vi "Dictionary Get Values.vi"(7 "lock dictionary? (FALSE)":bool, 8 "error in":errorcluster, 11 "dictionary":T1) -> (0 "error out":errorcluster, 2 "values":variant[](array[variant]), 3 "dictionary out":T1)   [LabVIEW 2009]
doc: "Returns all of the values within the dictionary. \n\n<B>lock dictionary</B> will lock the dictionary, preventing dictionary modifications until it is unlocked. Locking a dictionary is useful when the values of keys store compound data, which might be modified in multiple locations. The dictionary may be unlocked using the <B>unlock dictionary</B> input of the <B>Update Dictionary</B> function."
uses:
  Dictionary Object RefNum.ctl
  Dictionary Object RefNum - Enum.ctl
panel:
  # "Dictionary Get Values.vi\n\nReturns all of the values within the dictionary. \n\nPlease visit http://www.OpenG.org to learn about the\nOpen Source LabVIEW software movement.\n\nNOTICE -- YOU MUST LEAVE THIS NOTICE IN PLACE.  PER THE TERMS OF THE LICENSE BELOW, YOU MAY SUBLICENSE THIS SOFTWARE \nIN ANY WAY THAT DOES NOT CONFLICT WITH THIS LICENSE.\n\n### BSD License (http://www.opensource.org/licenses/bsd-license.php) Begin ###\n \nCopyright (c) 2005, Jim Kring <jim@jimkring.com>\n\nAll rights reserved.\n\nRedistribution and use in source and binary forms, with or without modification, are permitted provided that the following conditions are met:\n\n    * Redistributions of source code must retain the above copyright notice, this list of conditions and the following disclaimer.\n    * Redistributions in binary form must reproduce the above copyright notice, this list of conditions and the following disclaimer in the \n       documentation and/or other materials provided with the distribution.\n    * Neither the name of SciWare, James Kring, Inc., nor the names of its contributors may be used to endorse or promote products derived \n       from this software without specific prior written permission.\n\nTHIS SOFTWARE IS PROVIDED BY THE COPYRIGHT HOLDERS AND CONTRIBUTORS \"AS IS\" AND ANY EXPRESS OR IMPLIED WARRANTIES, \nINCLUDING, BUT NOT LIMITED TO, THE IMPLIED WARRANTIES OF MERCHANTABILITY AND FITNESS FOR A PARTICULAR PURPOSE ARE \nDISCLAIMED. IN NO EVENT SHALL THE COPYRIGHT OWNER OR CONTRIBUTORS BE LIABLE FOR ANY DIRECT, INDIRECT, INCIDENTAL,\n SPECIAL, EXEMPLARY, OR CONSEQUENTIAL DAMAGES (INCLUDING, BUT NOT LIMITED TO, PROCUREMENT OF SUBSTITUTE GOODS OR \nSERVICES; LOSS OF USE, DATA, OR PROFITS; OR BUSINESS INTERRUPTION) HOWEVER CAUSED AND ON ANY THEORY OF LIABILITY, \nWHETHER IN CONTRACT, STRICT LIABILITY, OR TORT (INCLUDING NEGLIGENCE OR OTHERWISE) ARISING IN ANY WAY OUT OF THE USE \nOF THIS SOFTWARE, EVEN IF ADVISED OF THE POSSIBILITY OF SUCH DAMAGE.\n\n### BSD License End ###"
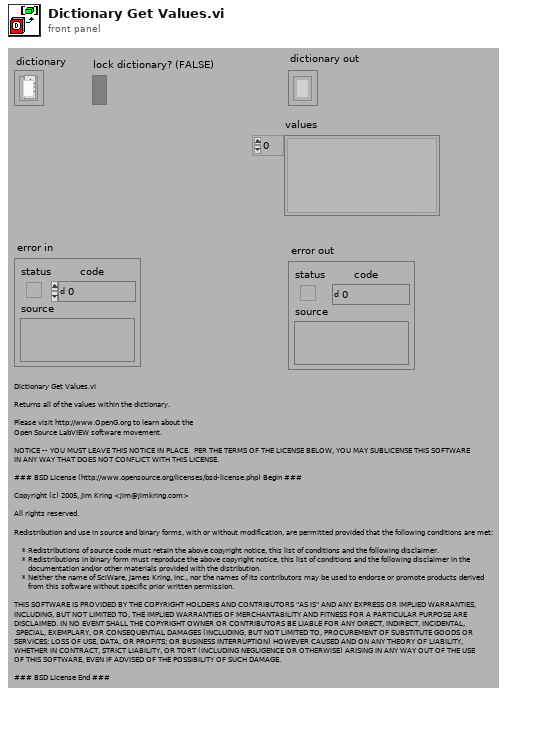
[diagram p1: front panel]
types:
  T1 = typedef "Dictionary Object RefNum.ctl" = refnum<k1>
  T2 = typedef "Dictionary Data.ctl" = cluster{"keys":variant[], "values":variant[]}
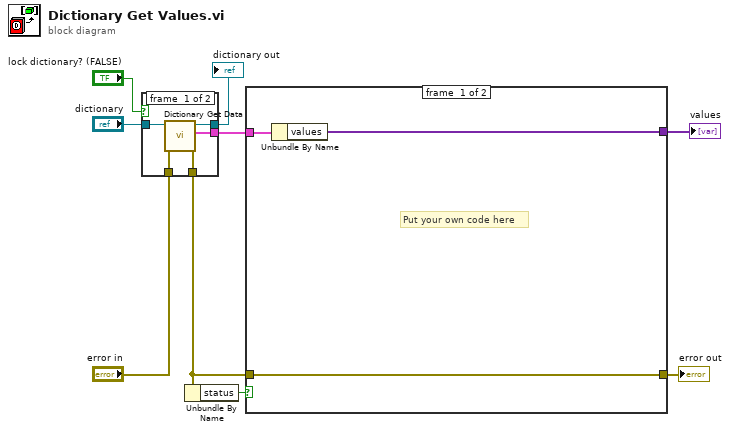
[diagram p0: block diagram]
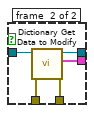
[diagram p2: hidden frame]
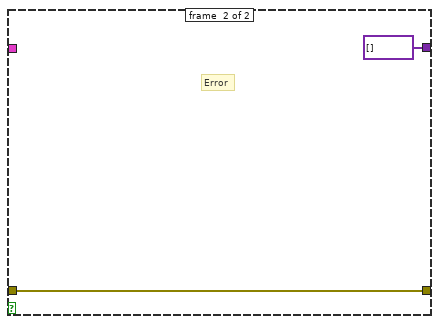
[diagram p3: hidden frame]
diagram:
  n1 = case shown="True" "lock dictionary? (FALSE)" {
    tunnel: [w14 w17] -> w3
    tunnel: "error in" -> [w13 w19]
    tunnel: [w12 w18] -> w4
    tunnel: [w11 w15] -> w2
    tunnel: "dictionary" -> [w10 w16]
    frame #0 {
      n2 = call "Dictionary Get Data.vi"("error in (no error)"=w13, "Object RefNum"=w10) -> ("error out"=w12:errorcluster, "Data out"=w14:T2, "Dup Object RefNum"=w11:T1)  [unwired: 7 in]
    }
    frame #1 {
      n3 = call "Dictionary Get Data to Modify.vi"("error in (no error)"=w19, "Object RefNum"=w16) -> ("error out"=w18:errorcluster, "Data out"=w17:T2, "Dup Object RefNum"=w15:T1)  [unwired: 6 in, 1 out]
    }
  }
  "dictionary out" <- w2
  n4 = Unbundle By Name(w4) -> ("status"=w9:bool)
  n5 = case shown="False" w9 {
    tunnel: w4 -> [w21 w24]
    tunnel: [w21 w24] -> w8
    tunnel: w3 -> [w22 _]
    tunnel: [w20 variant[] [] ("keys")] -> w7
    frame #0 {
      # "Put your own code here"
      n6 = Unbundle By Name(w22) -> ("values"=w20:variant[])
    }
    frame #1 {
      # "Error"
    }
  }
  "error out" <- w8
  "values" <- w7
